vi "搜索文件.vi"() -> ()   [LabVIEW 2023]
panel:
  out "进度":u8(slide) scale=0.0..1.0
  out "VI 文件":string[](array[string])
  in  "Path":path
  # "在一个指定文件夹里列出所有VI文件 并且 显示 完成搜索进度"
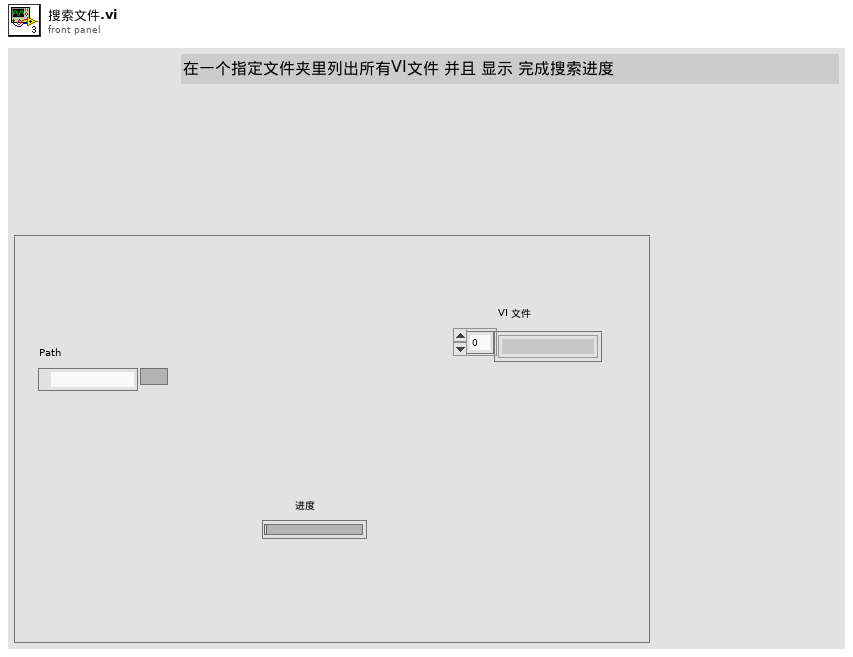
[diagram p1: front panel]
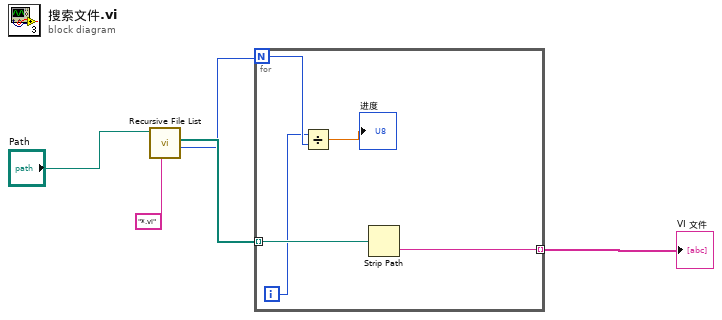
[diagram p0: block diagram]
diagram:
  n1 = call <vilib>:"Recursive File List.vi"("pattern"="*.vi", "Folder Path"="Path") -> ("Number of Files"=w1:i32, "All Files in Dir"=w3:path[])  [unwired: 5 in, 3 out]
  n2 = for {
    N: w1 -> [w8]
    tunnel: w3 -> [w10] mode=indexing
    tunnel: [w9] -> w2 mode=indexing
    i -> [w7]
    n3 = Divide(x=w7, y=w8) -> (x/y=→"进度":dbl)
    n4 = Strip Path(path=w10) -> (name=w9:string)  [unwired: 1 out]
  }
  "VI 文件" <- w2
